vi "GyroSpinning.vi"(11 "Angle":i32) -> ()   [LabVIEW 2015]
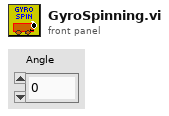
[diagram p1: front panel]
types:
  T1 = typedef "WPI_GyroDevRef.ctl" = cluster{"DevStatus":errorcluster, "Analog Module":T2, "Analog Channel":T3, "Offset":dbl, "Gain (VoltsPerDegree/Second)":dbl}
  T2 = typedef "FPGA_TypedefAnalogModule.ctl" = enum16{"Analog Module 1", "Analog Module 2"}
  T3 = typedef "FPGA_AIChannel.ctl" = enum8{"AI 1", "AI 2", "AI 3", "AI 4", "AI 5", "AI 6", "AI 7", "AI 8", "Invalid"}
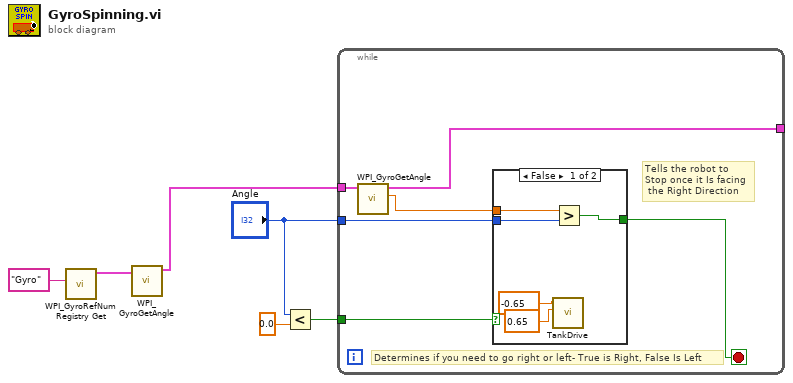
[diagram p0: block diagram]
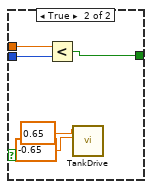
[diagram p2: hidden frame]
diagram:
  n1 = call <vilib>:"WPI_GyroRefNum Registry Get.vi"("refnum name"="Gyro") -> ("GyroDevRef"=w5:T1)  [unwired: 9 in, 1 out]
  n2 = call <vilib>:"WPI_GyroGetAngle.vi"("GyroDevRef"=w5) -> ("GyroDevRef"=w6:T1)  [unwired: 7 in, 3 out]
  n3 = Less?(x="Angle", y=0.0) -> (x < y?=w2:bool)
  n4 = while {
    tunnel: w6 -> [w12]
    tunnel: [w9] -> _
    tunnel: "Angle" -> [w8]
    tunnel: w2 -> [w7]
    stop <- w10 stop-if-true
    # "Tells the robot to \nStop once it Is facing\n the Right Direction"
    # "Determines if you need to go right or left- True is Right, False Is Left"
    n5 = call <vilib>:"WPI_GyroGetAngle.vi"("GyroDevRef"=w12) -> ("Angle"=w11:dbl, "GyroDevRef"=w9:T1)  [unwired: 7 in, 2 out]
    n6 = case shown="False" w7 {
      tunnel: w11 -> [w17 w22]
      tunnel: [w16 w21] -> w10
      tunnel: w8 -> [w13 w18]
      frame False {
        n7 = call "TankDrive.vi"("right"=0.65, "left"=-0.65) -> ()  [unwired: 10 in]
        n8 = Greater?(x=w17, y=w13) -> (0:w16:bool)
      }
      frame True {
        n9 = Less?(x=w22, y=w18) -> (x < y?=w21:bool)
        n10 = call "TankDrive.vi"("right"=-0.65, "left"=0.65) -> ()  [unwired: 10 in]
      }
    }
  }
